vi "GEN_Delete Same Element in array.vi"(10 "data in":string[](array[string])) -> (2 "data out":string[](array[string]))   [LabVIEW 2016]
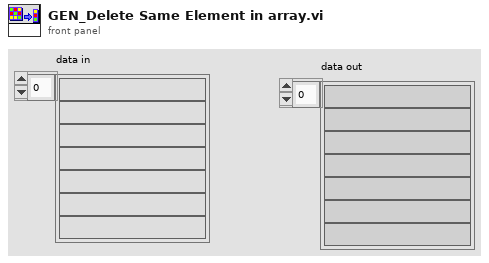
[diagram p1: front panel]
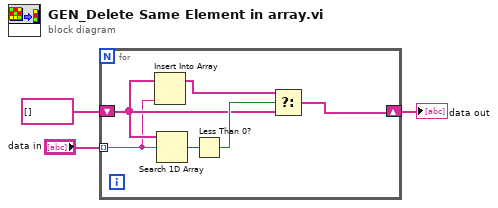
[diagram p0: block diagram]
diagram:
  n1 = for {
    tunnel: "data in" -> [w6] mode=indexing
    shift-right: [w4] -> w1
    shift-left: string[] [] ("data in") -> [w7]
    n2 = Insert Into Array(array=w7, new element=w6) -> (w5:string[])  [unwired: 1 in]
    n3 = Search 1D Array(1D array=w7, element=w6) -> (index of element=w9:i32)  [unwired: 1 in]
    n4 = Less Than 0?(x=w9) -> (x < 0?=w8:bool)
    n5 = Select(t=w5, s=w8, f=w7) -> (s? t:f=w4:string[])
  }
  "data out" <- w1
